vi "FTW-CodeGen-GetTerms4.vi"(0 "State In":T2, 5 "XRef":refnum<vi>) -> (4 "Terms":T1(array[cluster]))   [LabVIEW 2014, in "FTW-Array-Shuffle.xnode"]
uses:
  FTW-Array-Shuffle.xnode
  FTW-CodeGen-State.ctl
panel:
  # "Inputs"
  # "Outputs"
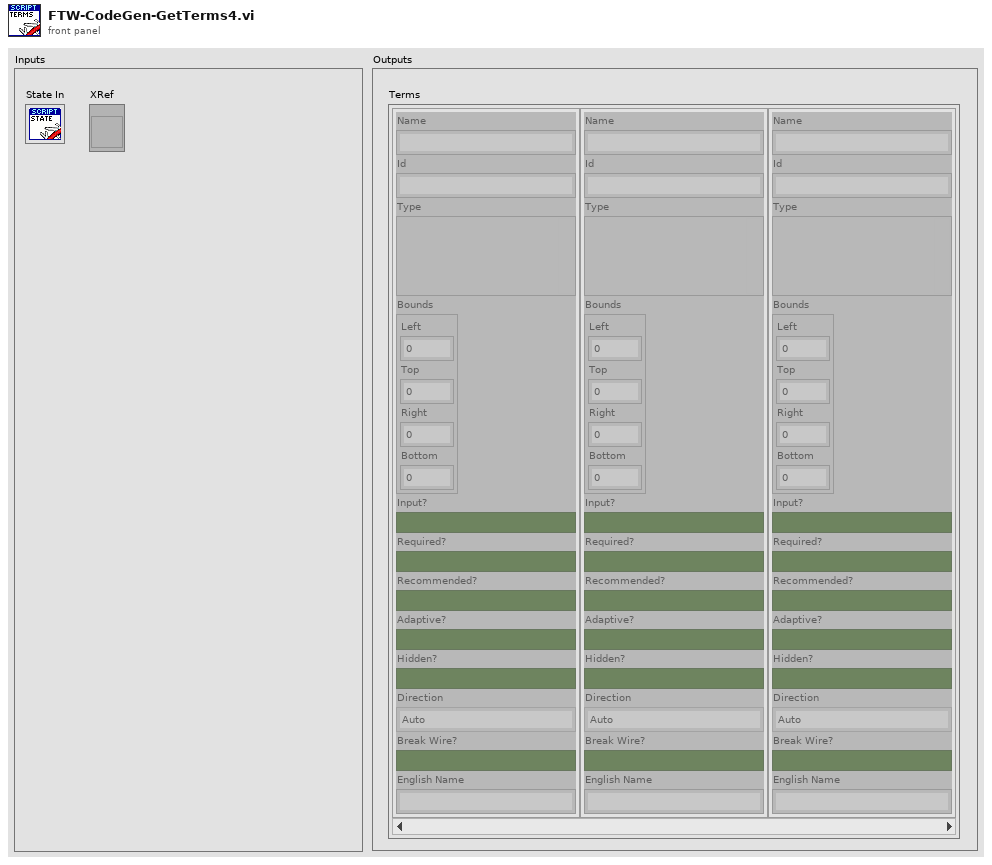
[diagram p1: front panel]
types:
  T1 = cluster{"Name":string, "Id":string, "Type":variant, "Bounds":cluster{"Left":i32, "Top":i32, "Right":i32, "Bottom":i32}, "Input?":bool, "Required?":bool, "Recommended?":bool, "Adaptive?":bool, "Hidden?":bool, "Direction":enum32{"Auto", "Up", "Down", "Left", "Right", "Center"}, "Break Wire?":bool, "English Name":string}[]
  T2 = typedef "FTW-Array-Shuffle.xnode/FTW-CodeGen-State.ctl" = cluster{"Dummy":string}
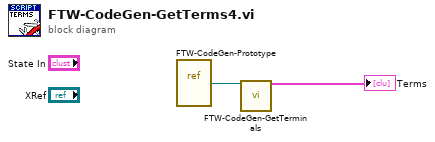
[diagram p0: block diagram]
diagram:
  n1 = vi-ref "FTW-CodeGen-Prototype.vi"() -> (w2:refnum<vi>)
  n2 = call "FTW-CodeGen-GetTerminals.vi"("PrototypeVI"=w2) -> ("Terms"=→"Terms":T1)  [unwired: 13 in, 1 out]
